vi "#9.vi"(0 "System no.":i32=1 min=1 max=4 step=1, 5 "error in":errorcluster) -> (14 "WG running?":bool[](array[boolean]), 19 "error out":errorcluster)   [LabVIEW 2020]
doc: "Polls to determine whether a wave generator is running for any of the connected axes by sending the single ASCII character 9. Connected axes are read from Global2.vi and displayed on the front panel for assignment.\n\nC-843: #9 polls the state of the User Profile mode."
panel:
  out "WaveGenerators":string[](array[string])
  in  "Read WG IDs?":bool
  out "Connected axes":string[](array[string])
  # "Polls to determine whether a wave generator is running for any of the connected axes."
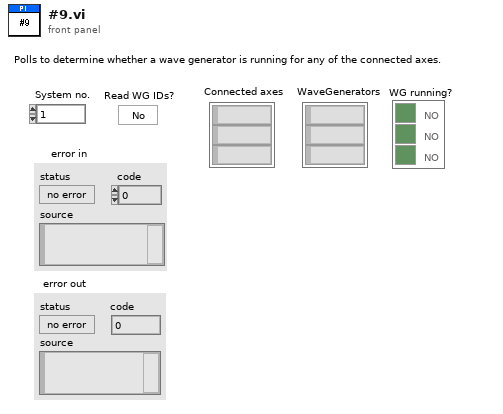
[diagram p1: front panel]
types:
  T1 = enum16{"Disable error check", "Force error check", "Use global settings"}
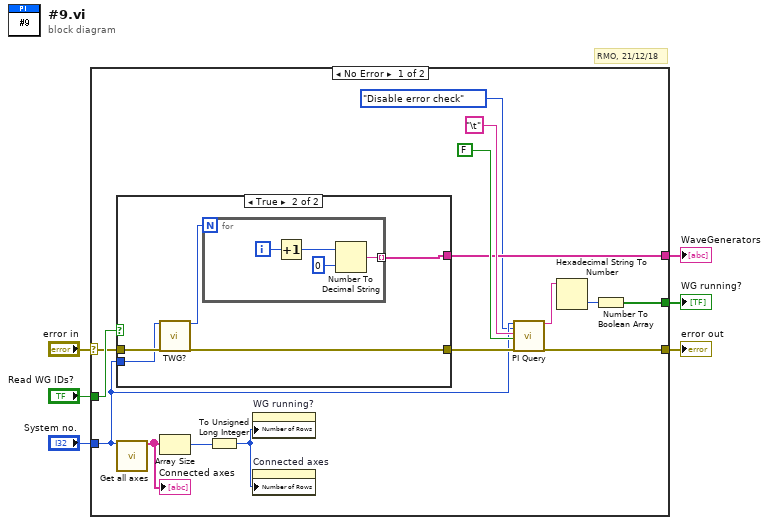
[diagram p0: block diagram]
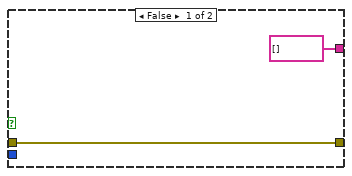
[diagram p2: hidden frame]
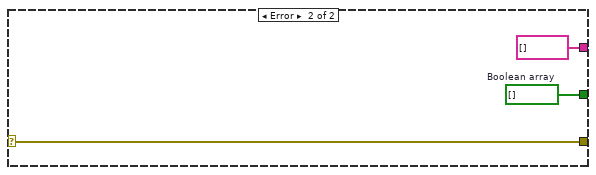
[diagram p3: hidden frame]
diagram:
  # "RMO, 21/12/18"
  n1 = case shown="No Error" "error in" {
    selector: "error in" -> [w10 w35]
    tunnel: [w19 w34] -> w6
    tunnel: [w7 w35] -> w5
    tunnel: [w14 string[] []] -> w4
    tunnel: "Read WG IDs?" -> [w12 _]
    tunnel: "System no." -> [w11 _]
    frame No Error {
      n2 = case shown="True" w12 {
        tunnel: [string[] [] w27] -> w14
        tunnel: w10 -> [w23 w26]
        tunnel: [w23 w25] -> w13
        tunnel: w11 -> [_ w24]
        frame False {
        }
        frame True {
          n3 = call "TWG?.vi"("System no."=w24, "error in"=w26) -> ("Number of wave generators"=w28:i32, "error out"=w25:errorcluster)  [unwired: 16 out]
          n4 = for {
            N: w28 -> [_]
            tunnel: [w29] -> w27 mode=indexing
            i -> [w32]
            n5 = Increment(x=w32) -> (x+1=w31:i32)
            n6 = Number To Decimal String(number=w31, width (-)=i16 0) -> (decimal integer string=w29:string)
          }
        }
      }
      n7 = call "Get all axes.vi"("System no."=w11) -> ("Conn. Axes"=w16:string[])  [unwired: 18 out]
      "Connected axes" <- w16
      n8 = Array Size(array=w16) -> (size(s)=w18:i32)
      n9 = To Unsigned Long Integer(number=w18) -> (unsigned 32bit integer=w15:u32)
      n10 = property on="WG running?" class="Arr (strict)"("Number of Rows"=w15) -> ()  [unwired: 2 in, 2 out]
      n11 = property on="Connected axes" class="Arr (strict)"("Number of Rows"=w15) -> ()  [unwired: 2 in, 2 out]
      n12 = call "PI Query.vi"("System no."=w11, "Error check settings"=T1."Disable error check", "String to send"="\t", "Attach termination char.?"=FALSE ("Attach Linefeed?"), "error in"=w13) -> ("String read"=w8:string, "error out"=w7:errorcluster)  [unwired: 2 in, 11 out]
      n13 = Hexadecimal String To Number(string=w8) -> (number=w17:u32)  [unwired: 3 out]
      n14 = Number To Boolean Array(number=w17) -> (Boolean array=w19:bool[])
    }
    frame Error {
      w34 = bool[] []  # Boolean array
    }
  }
  "error out" <- w5
  "WG running?" <- w6
  "WaveGenerators" <- w4
